vi "DAQexit(allmethods).vi"(8 "error in":errorcluster, 10 "Parameters":T1, 11 "INITout":refnum<class "RADEBase.lvclass">) -> (0 "error out":errorcluster)   [LabVIEW 2014]
uses:
  <userlib>/_RADE/RIO/RADEBase/classes/RADEBase/RADEBase.lvclass
  <userlib>/_RADE/RIO/JAPC/classes/JSubscribe/JSubscribe.lvclass
  <userlib>/_RADE/RIO/CMW/classes/CMWSubscribe/CMWSubscribe.lvclass
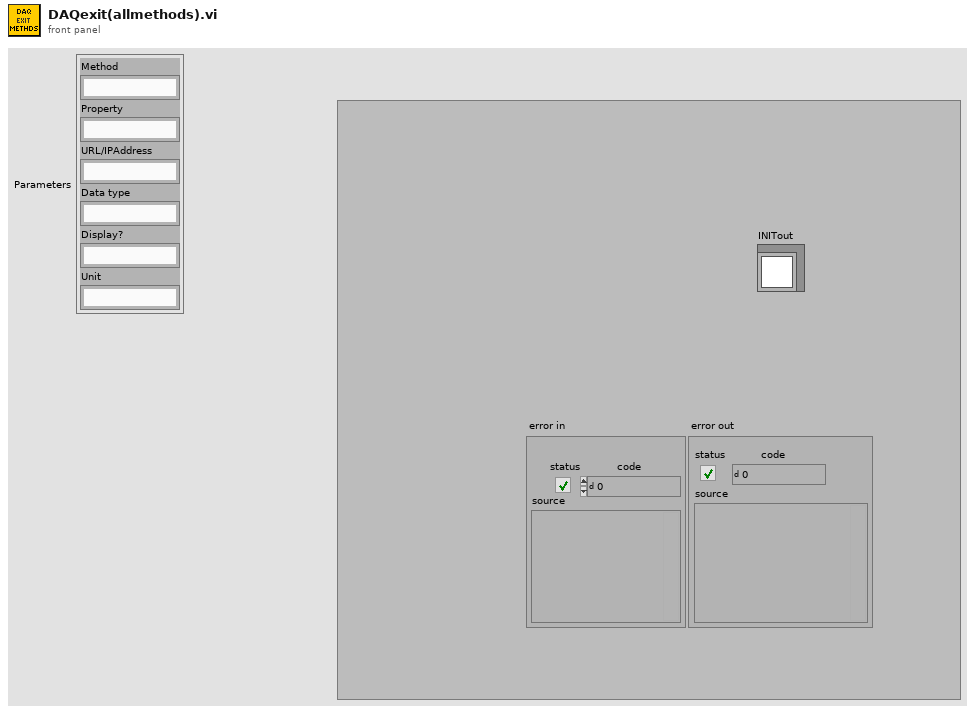
[diagram p1: front panel]
types:
  T1 = cluster{"Method":string, "Property":string, "URL/IPAddress":string, "Data type":string, "Display?":string, "Unit":string}
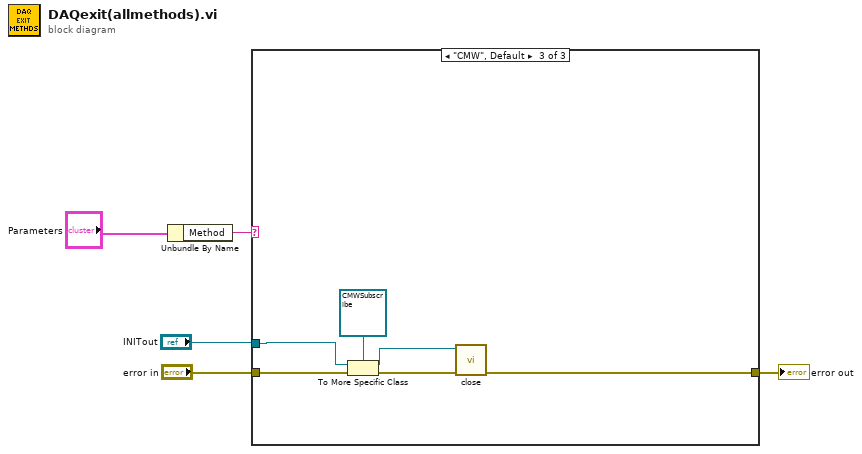
[diagram p0: block diagram]
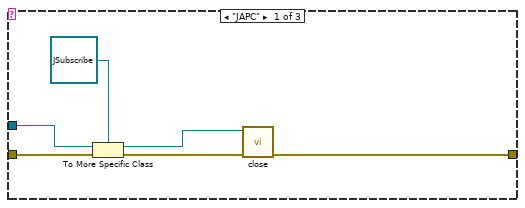
[diagram p2: hidden frame]
diagram:
  n1 = Unbundle By Name("Parameters") -> ("Method"=w3:string)
  n2 = case shown="\"CMW\", Default" w3 {
    tunnel: "error in" -> [w7 w12 w14]
    tunnel: [w11 w12 w18] -> w4
    tunnel: "INITout" -> [w10 _ w16]
    frame "JAPC" {
      n3 = To More Specific Class(target class=refnum<class "JSubscribe.lvclass"> refnum ("Object out"), reference=w10, error in=w7) -> (specific class reference=w8:refnum<class "JSubscribe.lvclass">, error out=w6:errorcluster)
      n4 = call-dynamic "close.vi"("error in (no error)"=w6, "Object in"=w8) -> ("error out"=w11:errorcluster)  [unwired: 9 in]
    }
    frame "PLC" {
    }
    frame "CMW", Default {
      n5 = To More Specific Class(target class=refnum<class "CMWSubscribe.lvclass"> refnum ("CMWout"), reference=w16, error in=w14) -> (specific class reference=w15:refnum<class "CMWSubscribe.lvclass">, error out=w13:errorcluster)
      n6 = call-dynamic "close.vi"("error in (no error)"=w13, "Object in"=w15) -> ("error out"=w18:errorcluster)  [unwired: 9 in]
    }
  }
  "error out" <- w4
